vi "FormatMessageTXT.vi"(0 "reference in":refnum<class "TelegramBOT.lvclass">, 2 "Text":string, 5 "error in (no error)":errorcluster) -> (14 "reference out":refnum<class "TelegramBOT.lvclass">, 16 "MsgTxt":string, 19 "error out":errorcluster)   [LabVIEW 2014, in "TelegramBOT.lvclass"]
uses:
  TelegramBOT.lvclass
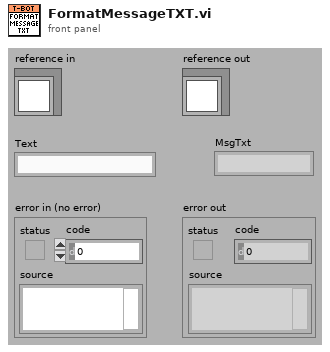
[diagram p1: front panel]
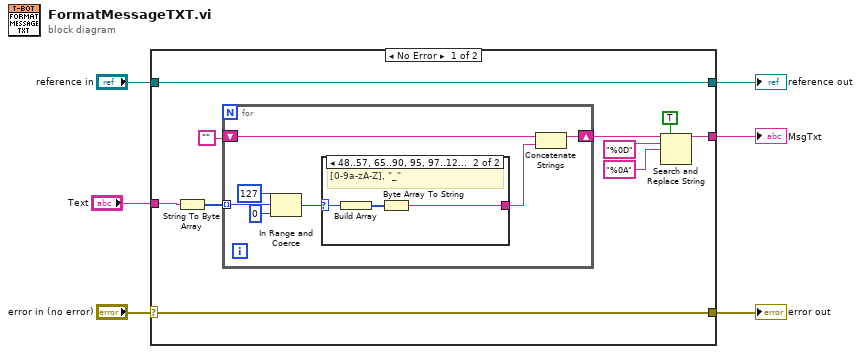
[diagram p0: block diagram]
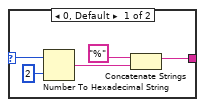
[diagram p2: hidden frame]
diagram:
  n1 = case shown="No Error" "error in (no error)" {
    selector: "error in (no error)" -> [w15 w33]
    tunnel: [w15 w33] -> w5
    tunnel: [w16 w32] -> w3
    tunnel: "reference in" -> [w16 w32]
    tunnel: "Text" -> [w8 _]
    tunnel: [w7 _] -> w1
    frame No Error {
      n2 = String To Byte Array(string=w8) -> (unsigned byte array=w9:u8[])
      n3 = for {
        tunnel: w9 -> [w20] mode=indexing
        shift-right: [w21] -> w13
        shift-left: "" -> [w22]
        n4 = In Range and Coerce(upper limit=u8 127, x=w20, lower limit=u8 0) -> (coerced(x)=w19:u8)  [unwired: 1 out]
        n5 = case shown="48..57, 65..90, 95, 97..122" w19 {
          selector: w19 -> [w28 w31]
          tunnel: [w24 w29] -> w23
          frame 0, Default {
            n6 = Number To Hexadecimal String(1:i16 2 ("width (-)"), 2:w28) -> (0:w26:string)
            n7 = Concatenate Strings("%" ("string"), w26) -> (w24:string)
          }
          frame 48..57, 65..90, 95, 97..122 {
            # "[0-9a-zA-Z], \"_\""
            n8 = Build Array(w31) -> (w30:u8[])
            n9 = Byte Array To String(unsigned byte array=w30) -> (string=w29:string)
          }
        }
        n10 = Concatenate Strings(w22, w23) -> (w21:string)
      }
      n11 = Search and Replace String(replace all?=TRUE ("replace all? (F)"), input string=w13, search string="%0D", replace string="%0A" ("replace string (\"\")")) -> (result string=w7:string)  [unwired: 4 in, 3 out]
    }
    frame Error {
    }
  }
  "error out" <- w5
  "reference out" <- w3
  "MsgTxt" <- w1
